vi "data insert.vi"(8 "error in (no error)":errorcluster, 10 "运行模式":enum16{"维护模式", "常规模式"}(ring), 11 "modbus-data":T2) -> (0 "error out":errorcluster)   [LabVIEW 2016, in "SL1500-3G.lvlib"]
uses:
  SL1500-3G.lvlib
  Ctl/modbus output data.ctl
  <vilib>/addons/database/Auxilliary.llb/DB Tools Column Info.ctl
  <vilib>/addons/database/Auxilliary.llb/DB Tools DataTypes.ctl
  <vilib>/addons/database/NI_Database_API.lvlib
  <vilib>/Utility/VariantDataType/VariantType.lvlib
panel:
  in  "Total volume":T1={"时间"=timestamp(0 s since 1904-01-01), "测量模式"="水样测试", "数据类型"="N", "检测值"=0.0, "单位"="m3", "数据标识"="N", "因子编码"="e01204"}
  in  "Flow rate":T1={"时间"=timestamp(0 s since 1904-01-01), "测量模式"="水样测试", "数据类型"="N", "检测值"=0.0, "单位"="m3/s", "数据标识"="N", "因子编码"="e01203"}
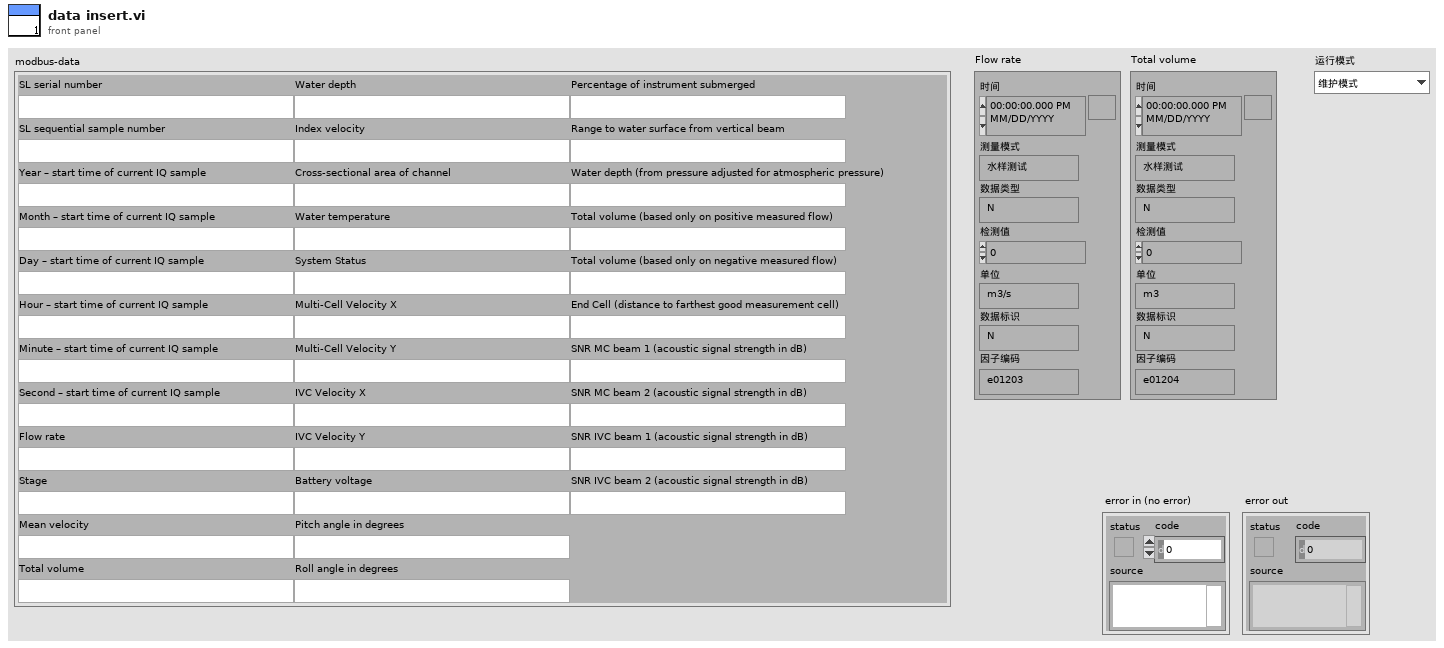
[diagram p1: front panel]
types:
  T1 = cluster{"时间":timestamp, "测量模式":string, "数据类型":string, "检测值":sgl, "单位":string, "数据标识":string, "因子编码":string}
  T2 = typedef "SL1500-3G.lvlib/modbus output data.ctl" = cluster{"SL serial number":dbl, "SL sequential sample number":dbl, "Year – start time of current IQ sample":dbl, "Month – start time of current IQ sample":dbl, "Day – start time of current IQ sample":dbl, "Hour – start time of current IQ sample":dbl, "Minute – start time of current IQ sample":dbl, "Second – start time of current IQ sample":dbl, "Flow rate":dbl, "Stage":dbl, "Mean velocity":dbl, "Total volume":dbl, "Water depth":dbl, "Index velocity":dbl, "Cross-sectional area of channel":dbl, "Water temperature":dbl, "System Status":dbl, "Multi-Cell Velocity X":dbl, "Multi-Cell Velocity Y":dbl, "IVC Velocity X":dbl, "IVC Velocity Y":dbl, "Battery voltage":dbl, "Pitch angle in degrees":dbl, "Roll angle in degrees":dbl, "Percentage of instrument submerged":dbl, "Range to water surface from vertical beam":dbl, "Water depth (from pressure adjusted for atmospheric pressure)":dbl, "Total volume (based only on positive measured flow)":dbl, "Total volume (based only on negative measured flow)":dbl, "End Cell (distance to farthest good measurement cell)":dbl, "SNR MC beam 1 (acoustic signal strength in dB)":dbl, "SNR MC beam 2 (acoustic signal strength in dB)":dbl, "SNR IVC beam 1 (acoustic signal strength in dB)":dbl, "SNR IVC beam 2 (acoustic signal strength in dB)":dbl}
  T3 = typedef "NI_Database_API.lvlib/DB Tools Column Info.ctl" = cluster{"column name":string, "data type":T4, "size":i32, "allow null?":bool}
  T4 = typedef "NI_Database_API.lvlib/DB Tools DataTypes.ctl" = enum16{"String", "Long (I32)", "Single (SGL)", "Double (DBL)", "Date/Time", "Binary"}
  T5 = typedef "VariantType.lvlib/Type.ctl" = enum8{"Invalid Type", "Void", "I8", "I16", "I32", "I64", "U8", "U16", "U32", "U64", "Single Float", "Double Float", "Extended Float", "Single Complex", "Double Complex", "Extended Complex", "Enum U8", "Enum U16", "Enum U32", "Enum U64", "Single Float With Unit", "Double Float With Unit", "Extended Float With Unit", "Single Complex with Unit", "Double Complex with Unit", "Extended Complex with Unit", "Boolean", "String", "Path", "Picture", "Tag", "Array", "Cluster", "Variant", "LV Variant", "Waveform", "Timestamp", "Digital Waveform", "Digital Data", "ExpressData", "Refnum", "External Data", "VI", "Poly VI", "LabVIEW Class Instance", "Fixed Point"}
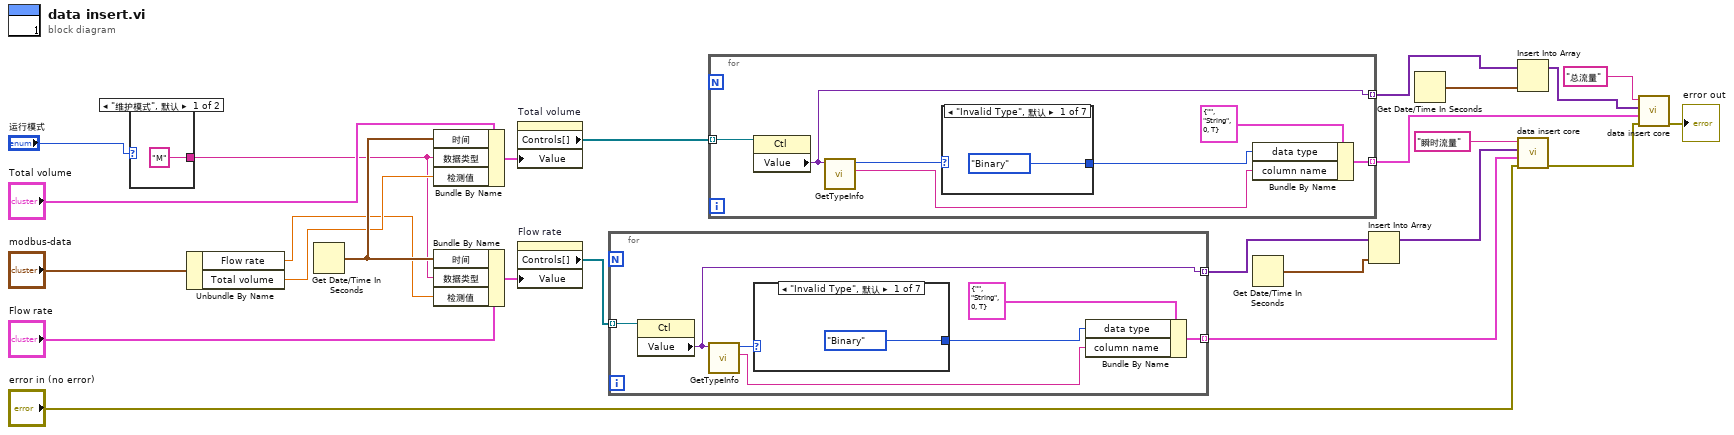
[diagram p0: block diagram]
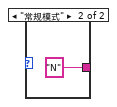
[diagram p2: hidden frame]
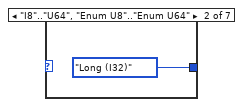
[diagram p3: hidden frame]
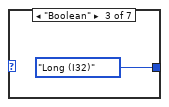
[diagram p4: hidden frame]
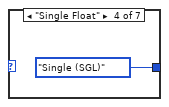
[diagram p5: hidden frame]
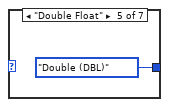
[diagram p6: hidden frame]
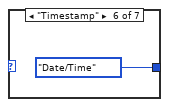
[diagram p7: hidden frame]
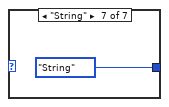
[diagram p8: hidden frame]
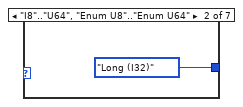
[diagram p9: hidden frame]
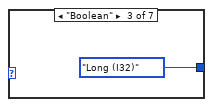
[diagram p10: hidden frame]
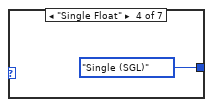
[diagram p11: hidden frame]
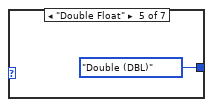
[diagram p12: hidden frame]
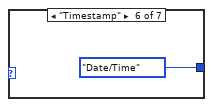
[diagram p13: hidden frame]
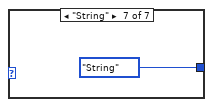
[diagram p14: hidden frame]
diagram:
  n1 = case shown="\"维护模式\", 默认" "运行模式" {
    tunnel: ["M" "N"] -> w1
    frame "维护模式", Default {
    }
    frame "常规模式" {
    }
  }
  n2 = Unbundle By Name("modbus-data") -> ("Flow rate"=w3:dbl, "Total volume"=w4:dbl)
  n3 = Get Date/Time In Seconds() -> (seconds since 1Jan1904=w5:timestamp)
  n4 = Bundle By Name(cluster="Total volume", "时间"=w5, "数据类型"=w1, "检测值"=w4) -> (w15:T1)
  n5 = Bundle By Name(cluster="Flow rate", "时间"=w5, "数据类型"=w1, "检测值"=w3) -> (w17:T1)
  n6 = property on="Total volume" class="Clust (严格)"("Value"=w15) -> ("Controls[]"=w14:refnum<vi>[])  [unwired: 2 in, 2 out]
  n7 = property on="Flow rate" class="Clust (严格)"("Value"=w17) -> ("Controls[]"=w18:refnum<vi>[])  [unwired: 2 in, 2 out]
  n8 = for {
    tunnel: w18 -> [w34] mode=indexing
    tunnel: [w28] -> w25 mode=indexing
    tunnel: [w29] -> w21 mode=indexing
    n9 = property class="Ctl"(reference=w34) -> ("Value"=w28:variant)  [unwired: 1 in, 2 out]
    n10 = call <vilib>:"GetTypeInfo.vi"("Variant"=w28) -> ("Name"=w32:string, "Type Enum"=w31:T5)  [unwired: 6 in, 3 out]
    n11 = case shown="\"Invalid Type\", 默认" w31 {
      tunnel: [DB_Tools_DataTypes."Binary" ("data type") DB_Tools_DataTypes."Long (I32)" ("data type") DB_Tools_DataTypes."Long (I32)" ("data type") DB_Tools_DataTypes."Single (SGL)" ("data type") DB_Tools_DataTypes."Double (DBL)" ("data type") DB_Tools_DataTypes."Date/Time" ("data type") DB_Tools_DataTypes."String" ("data type")] -> w30
      frame "Invalid Type", Default {
      }
      frame "I8".."U64", "Enum U8".."Enum U64" {
      }
      frame "Boolean" {
      }
      frame "Single Float" {
      }
      frame "Double Float" {
      }
      frame "Timestamp" {
      }
      frame "String" {
      }
    }
    n12 = Bundle By Name(cluster=T3 {"column name"="", "data type"=enum."String", "size"=0, "allow null?"=TRUE} ("column information"), "data type"=w30, "column name"=w32) -> (w29:T3)
  }
  n13 = for {
    tunnel: w14 -> [w48] mode=indexing
    tunnel: [w42] -> w9 mode=indexing
    tunnel: [w43] -> w12 mode=indexing
    n14 = property class="Ctl"(reference=w48) -> ("Value"=w42:variant)  [unwired: 1 in, 2 out]
    n15 = call <vilib>:"GetTypeInfo.vi"("Variant"=w42) -> ("Name"=w46:string, "Type Enum"=w45:T5)  [unwired: 6 in, 3 out]
    n16 = case shown="\"Invalid Type\", 默认" w45 {
      tunnel: [DB_Tools_DataTypes."Binary" ("data type") DB_Tools_DataTypes."Long (I32)" ("data type") DB_Tools_DataTypes."Long (I32)" ("data type") DB_Tools_DataTypes."Single (SGL)" ("data type") DB_Tools_DataTypes."Double (DBL)" ("data type") DB_Tools_DataTypes."Date/Time" ("data type") DB_Tools_DataTypes."String" ("data type")] -> w44
      frame "Invalid Type", Default {
      }
      frame "I8".."U64", "Enum U8".."Enum U64" {
      }
      frame "Boolean" {
      }
      frame "Single Float" {
      }
      frame "Double Float" {
      }
      frame "Timestamp" {
      }
      frame "String" {
      }
    }
    n17 = Bundle By Name(cluster=T3 {"column name"="", "data type"=enum."String", "size"=0, "allow null?"=TRUE} ("column information"), "data type"=w44, "column name"=w46) -> (w43:T3)
  }
  n18 = Get Date/Time In Seconds() -> (seconds since 1Jan1904=w24:timestamp)
  n19 = Insert Into Array(array=w25, new element=w24) -> (w23:variant[])  [unwired: 1 in]
  n20 = Get Date/Time In Seconds() -> (seconds since 1Jan1904=w10:timestamp)
  n21 = Insert Into Array(array=w9, new element=w10) -> (w11:variant[])  [unwired: 1 in]
  n22 = call "data insert core.vi"("error in (no error)"="error in (no error)", "column information"=w21, "data"=w23, "table"="瞬时流量") -> ("error out"=w8:errorcluster)  [unwired: 7 in]
  n23 = call "data insert core.vi"("error in (no error)"=w8, "column information"=w12, "data"=w11, "table"="总流量") -> ("error out"=→"error out":errorcluster)  [unwired: 7 in]
